vi "Apply Pretty Policy.vi"(9 "String":string, 11 "StringFormatter":refnum<class "StringFormatter.lvclass">) -> (1 "Pretty String":string, 3 "StringFormatter out":refnum<class "StringFormatter.lvclass">)   [LabVIEW 2013, in "OpenStringFormatter.lvlib" / "StringFormatter.lvclass"]
uses:
  StringFormatter.lvclass
  StringFormatter.lvclass/StringFormatter.ctl
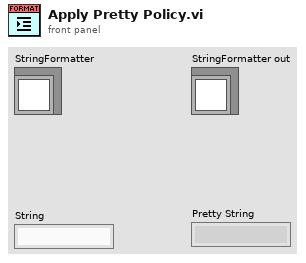
[diagram p1: front panel]
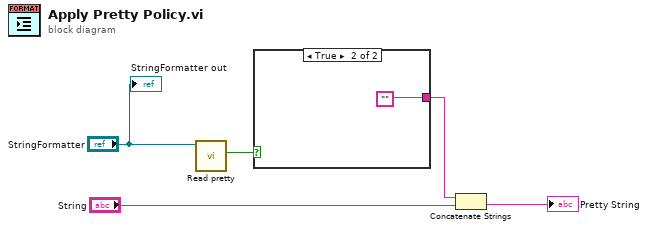
[diagram p0: block diagram]
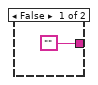
[diagram p2: hidden frame]
diagram:
  n1 = call "Read pretty.vi"("StringFormatter in"="StringFormatter") -> ("pretty"=w2:bool)  [unwired: 9 in, 1 out]
  n2 = case shown="True" w2 {
    tunnel: ["" ""] -> w3
    frame False {
    }
    frame True {
    }
  }
  n3 = Concatenate Strings(w3, "String") -> (→"Pretty String":string)
  "StringFormatter out" <- "StringFormatter"
